vi "SensorMetrix example.vi"() -> ()   [LabVIEW 2014]
uses:
  Que lib/Initialise.vi
  Que lib/Write.vi
  Lib/Read T3110.vi
  Lib/Read T2114.vi
  <vilib>/NI/Modbus Library/API/Master/Modbus Master.lvclass
  Que lib/Que lib.lvlib
  Lib/T3110 & T2114.lvlib
panel:
  in  "T2114 COM":refnum<visa-resource-name>
  out "Pressure Average, hPa":dbl
  in  "Stop Button":bool
  in  "T3110 COM":refnum<visa-resource-name>
  out "Temperature Average":dbl
  out "Humidity Average":dbl
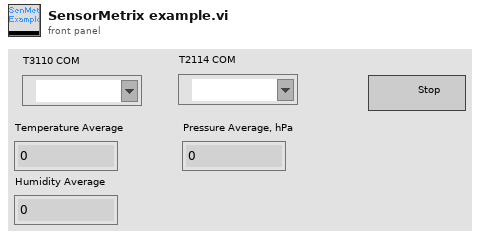
[diagram p1: front panel]
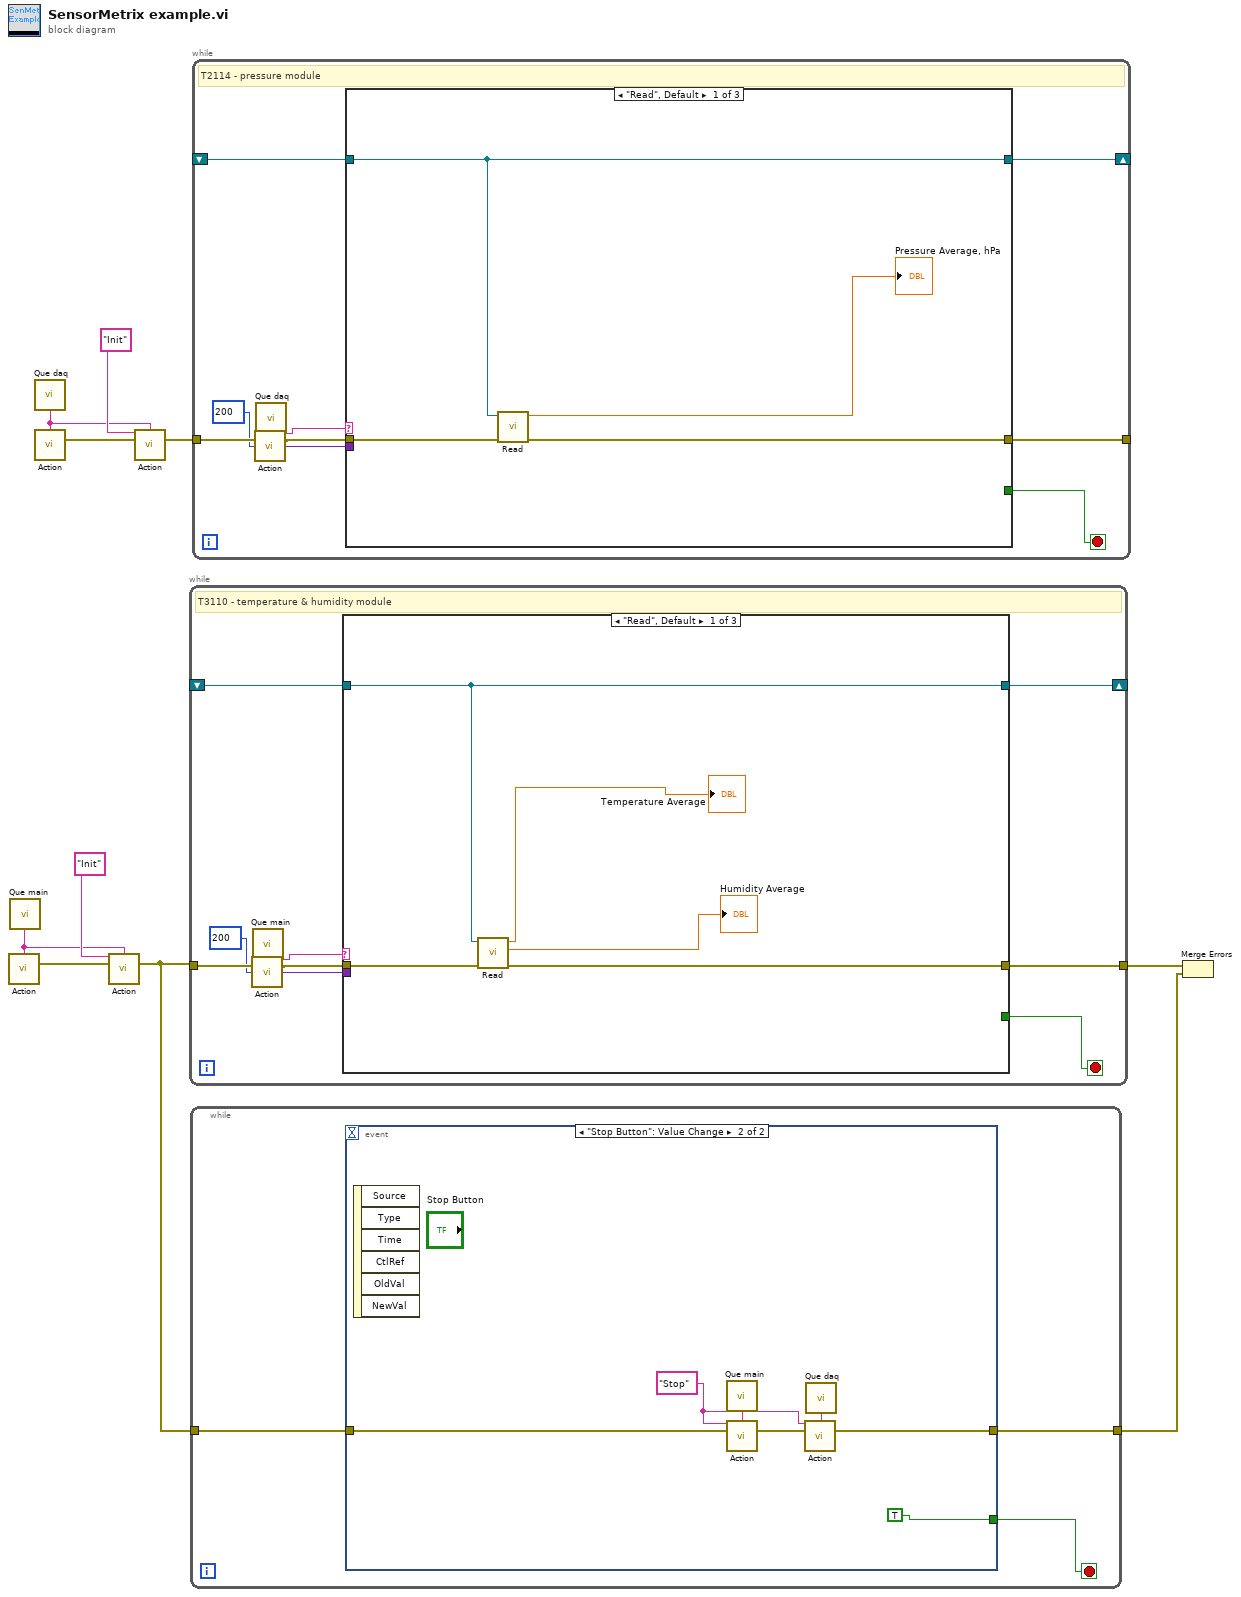
[diagram p0: block diagram]
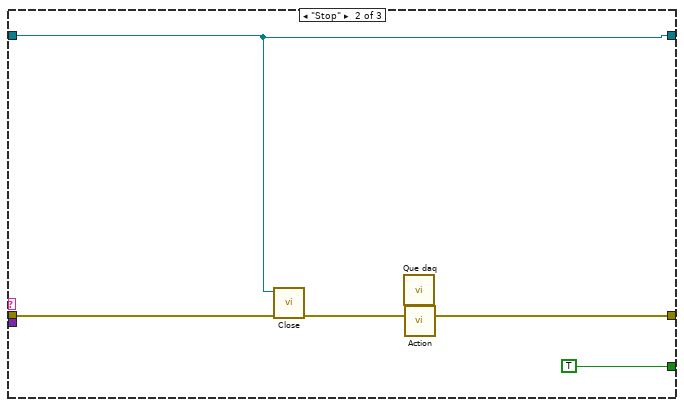
[diagram p2: hidden frame]
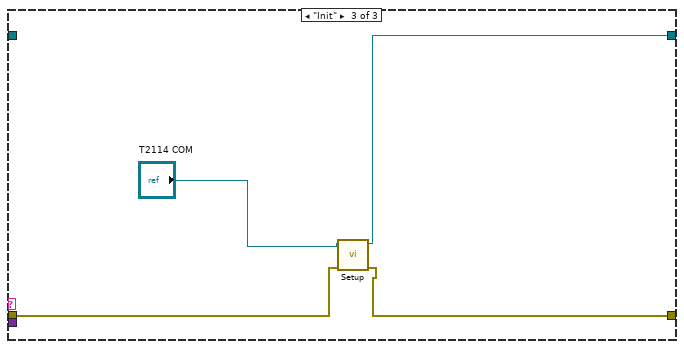
[diagram p3: hidden frame]
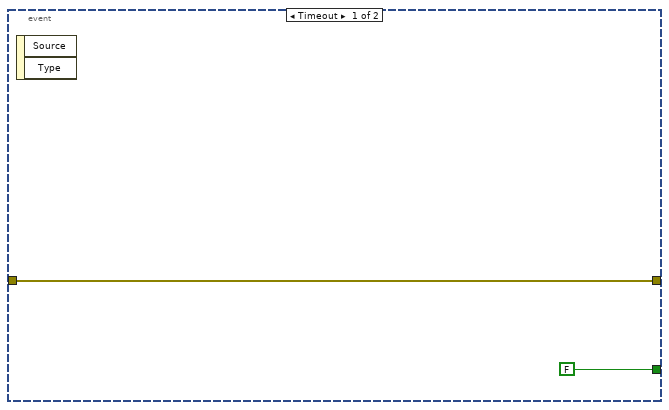
[diagram p4: hidden frame]
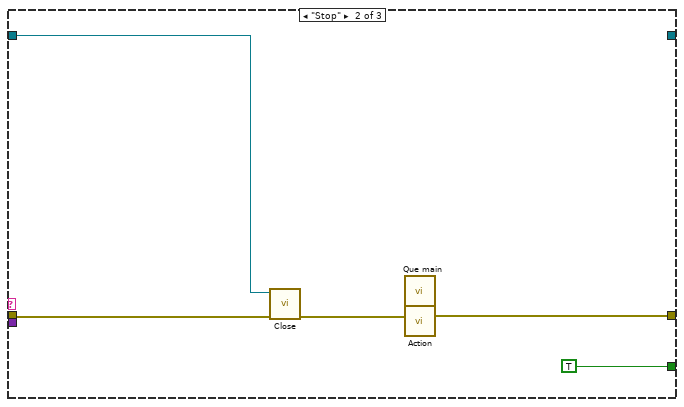
[diagram p5: hidden frame]
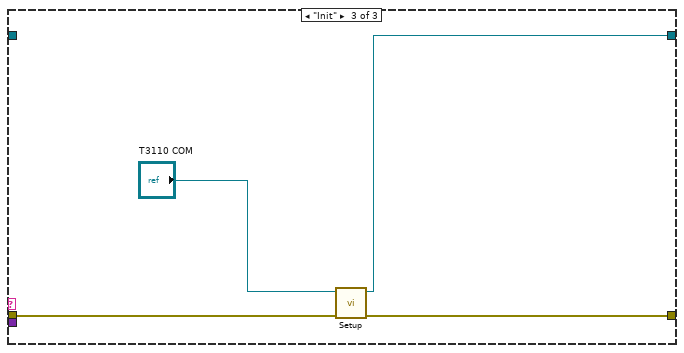
[diagram p6: hidden frame]
diagram:
  n1 = call "Que main.vi"() -> ("Que name"=w8:string)  [unwired: 15 in]
  n2 = call-poly "Action.vi"("Que name"=w8) -> ("error out"=w10:errorcluster)  [unwired: 14 in]
  n3 = call "Que daq.vi"() -> ("Que name"=w1:string)  [unwired: 15 in]
  n4 = call-poly "Action.vi"("Que name"=w1) -> ("error out"=w3:errorcluster)  [unwired: 14 in]
  n5 = call-poly "Action.vi"("Message"="Init" ("element"), "Que name"=w8, "error in"=w10) -> ("error out"=w7:errorcluster)  [unwired: 12 in]
  n6 = call-poly "Action.vi"("Message"="Init" ("element"), "Que name"=w1, "error in"=w3) -> ("error out"=w2:errorcluster)  [unwired: 12 in]
  n7 = while {
    tunnel: w7 -> [w15]
    shift-right: [w20] -> _
    shift-left: _ -> [w18]
    tunnel: [w19] -> w6
    stop <- w17 stop-if-true
    # "T3110 - temperature & humidity module"
    n8 = call "Que main.vi"() -> ("Que name"=w11:string)  [unwired: 15 in]
    n9 = call-poly "Action.vi"("Que name"=w11, "error in"=w15, "Timeout (default 2s)"=200 ("timeout in ms (-1)")) -> ("Message out"=w13:string, "error out"=w16:errorcluster, "Data"=w12:variant)  [unwired: 10 in]
    n10 = case shown="\"Read\", Default" w13 {
      tunnel: w16 -> [w25 w27 w35]
      tunnel: [w23 _ w32] -> w20
      tunnel: [w24 w30 w34] -> w19
      tunnel: w18 -> [w23 w26 _]
      tunnel: [_ TRUE _] -> w17
      tunnel: w12 -> [_ _ _]
      frame "Read", Default {
        n11 = call-poly "Read.vi"("error in"=w25, "Modbus master in"=w23) -> ("error out"=w24:errorcluster, "Humidity, %"=→"Humidity Average":dbl, "Temperature, deg C"=→"Temperature Average":dbl)  [unwired: 7 in]
      }
      frame "Stop" {
        n12 = call "Close.vi"("error in"=w27, "Modbus instance in"=w26) -> ("error out"=w28:errorcluster)  [unwired: 9 in]
        n13 = call "Que main.vi"() -> ("Que name"=w29:string)  [unwired: 15 in]
        n14 = call-poly "Action.vi"("Que name"=w29, "error in"=w28) -> ("error out"=w30:errorcluster)  [unwired: 13 in]
      }
      frame "Init" {
        n15 = call "Setup.vi"("error in"=w35, "Sensormetrix COM port"="T3110 COM") -> ("error out"=w34:errorcluster, "Modbus master out"=w32:refnum<class "Modbus Master.lvclass">)  [unwired: 8 in]
      }
    }
  }
  n16 = while {
    tunnel: w7 -> [w37]
    tunnel: [w36] -> w5
    stop <- w38 stop-if-true
    n17 = event shown="[1] \"Stop Button\": Value Change" {
      selector: _ -> [_ _]
      dyn-events: _ -> [_ _]
      timeout: _ -> [_ _]
      tunnel: [FALSE TRUE] -> w38
      tunnel: w37 -> [w39 w45]
      tunnel: [w39 w41] -> w36
      event Timeout {
        n18 = event-data() -> ()  [unwired: 1 in, 2 out]
      }
      event "Stop Button": Value Change {
        w43 = "Stop" ("Message")
        n19 = event-data() -> ()  [unwired: 1 in, 6 out]
        n20 = call "Que main.vi"() -> ("Que name"=w47:string)  [unwired: 15 in]
        n21 = call-poly "Action.vi"("Message"=w43, "Que name"=w47, "error in"=w45) -> ("error out"=w44:errorcluster)  [unwired: 12 in]
        n22 = call "Que daq.vi"() -> ("Que name"=w42:string)  [unwired: 15 in]
        n23 = call-poly "Action.vi"("Message"=w43, "Que name"=w42, "error in"=w44) -> ("error out"=w41:errorcluster)  [unwired: 12 in]
      }
    }
  }
  n24 = while {
    tunnel: w2 -> [w52]
    shift-right: [w57] -> _
    shift-left: _ -> [w55]
    tunnel: [w56] -> _
    stop <- w54 stop-if-true
    # "T2114 - pressure module"
    n25 = call "Que daq.vi"() -> ("Que name"=w48:string)  [unwired: 15 in]
    n26 = call-poly "Action.vi"("Que name"=w48, "error in"=w52, "Timeout (default 2s)"=200 ("timeout in ms (-1)")) -> ("Message out"=w50:string, "error out"=w53:errorcluster, "Data"=w49:variant)  [unwired: 10 in]
    n27 = case shown="\"Read\", Default" w50 {
      tunnel: w53 -> [w61 w65 w70]
      tunnel: [w59 w62 w68] -> w57
      tunnel: [w60 w66 w71] -> w56
      tunnel: w55 -> [w59 w62 _]
      tunnel: [_ TRUE _] -> w54
      tunnel: w49 -> [_ _ _]
      frame "Read", Default {
        n28 = call-poly "Read.vi"("error in"=w61, "Modbus master in"=w59) -> ("error out"=w60:errorcluster, "Ambient Pressure, hPa"=→"Pressure Average, hPa":dbl)  [unwired: 8 in]
      }
      frame "Stop" {
        n29 = call "Close.vi"("error in"=w65, "Modbus instance in"=w62) -> ("error out"=w64:errorcluster)  [unwired: 9 in]
        n30 = call "Que daq.vi"() -> ("Que name"=w63:string)  [unwired: 15 in]
        n31 = call-poly "Action.vi"("Que name"=w63, "error in"=w64) -> ("error out"=w66:errorcluster)  [unwired: 13 in]
      }
      frame "Init" {
        n32 = call "Setup.vi"("error in"=w70, "Sensormetrix COM port"="T2114 COM") -> ("error out"=w71:errorcluster, "Modbus master out"=w68:refnum<class "Modbus Master.lvclass">)  [unwired: 8 in]
      }
    }
  }
  n33 = Merge Errors(w6, w5) -> ()  [unwired: 1 out]
